vi "Master Target.vi"() -> ()   [LabVIEW 2011]
uses:
  Common/controls/Grips Buttons.ctl
  Common/classes/PXI/PXI.lvclass
  Common/classes/GripsMaster/GripsMaster.lvclass
  Common/controls/Task Definition.ctl
  Common/controls/Task Types.ctl
  Common/labview_msgs/sensor_msgs/JointState.ctl
panel:
  in  "Slave IP":string="138.100.76.41"
  out "UDP Status":errorcluster
  in  "Write Port":u16=5555
  out "Grips Buttons":T1
  in  "Stop":bool
  out "Controller Status":errorcluster
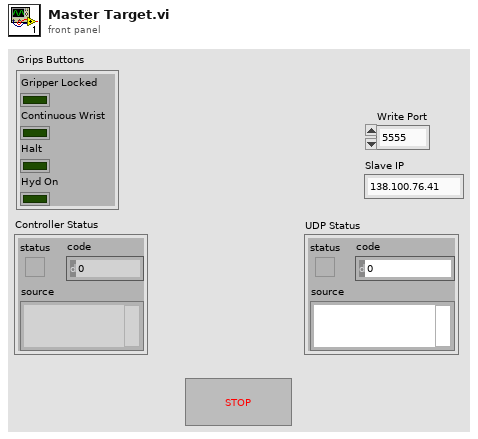
[diagram p1: front panel]
types:
  T1 = typedef "Grips Buttons.ctl" = cluster{"Gripper Locked":bool, "Continuous Wrist":bool, "Halt":bool, "Hyd On":bool}
  T2 = typedef "Task Definition.ctl" = cluster{"task_type":T3, "names":string[], "physical channels":tag, "min_value":dbl, "max_value":dbl, "task_number":i32}
  T3 = typedef "Task Types.ctl" = enum16{"Analog Input", "Analog Output", "Digital Input", "Digital Output"}
  T4 = typedef "Digital Values.ctl" = cluster{"names":string[], "values":bool[]}
  T5 = typedef "Analog Values.ctl" = cluster{"names":string[], "values":dbl[]}
  T6 = enum16{"big-endian, network order", "native, host order", "little-endian"}
  T7 = typedef "JointState.ctl" = cluster{"header":cluster{"seq":u32, "stamp":cluster{"sec":i32, "nsec":i32}, "frame_id":string}, "name":string[], "position":dbl[], "velocity":dbl[], "effort":dbl[]}
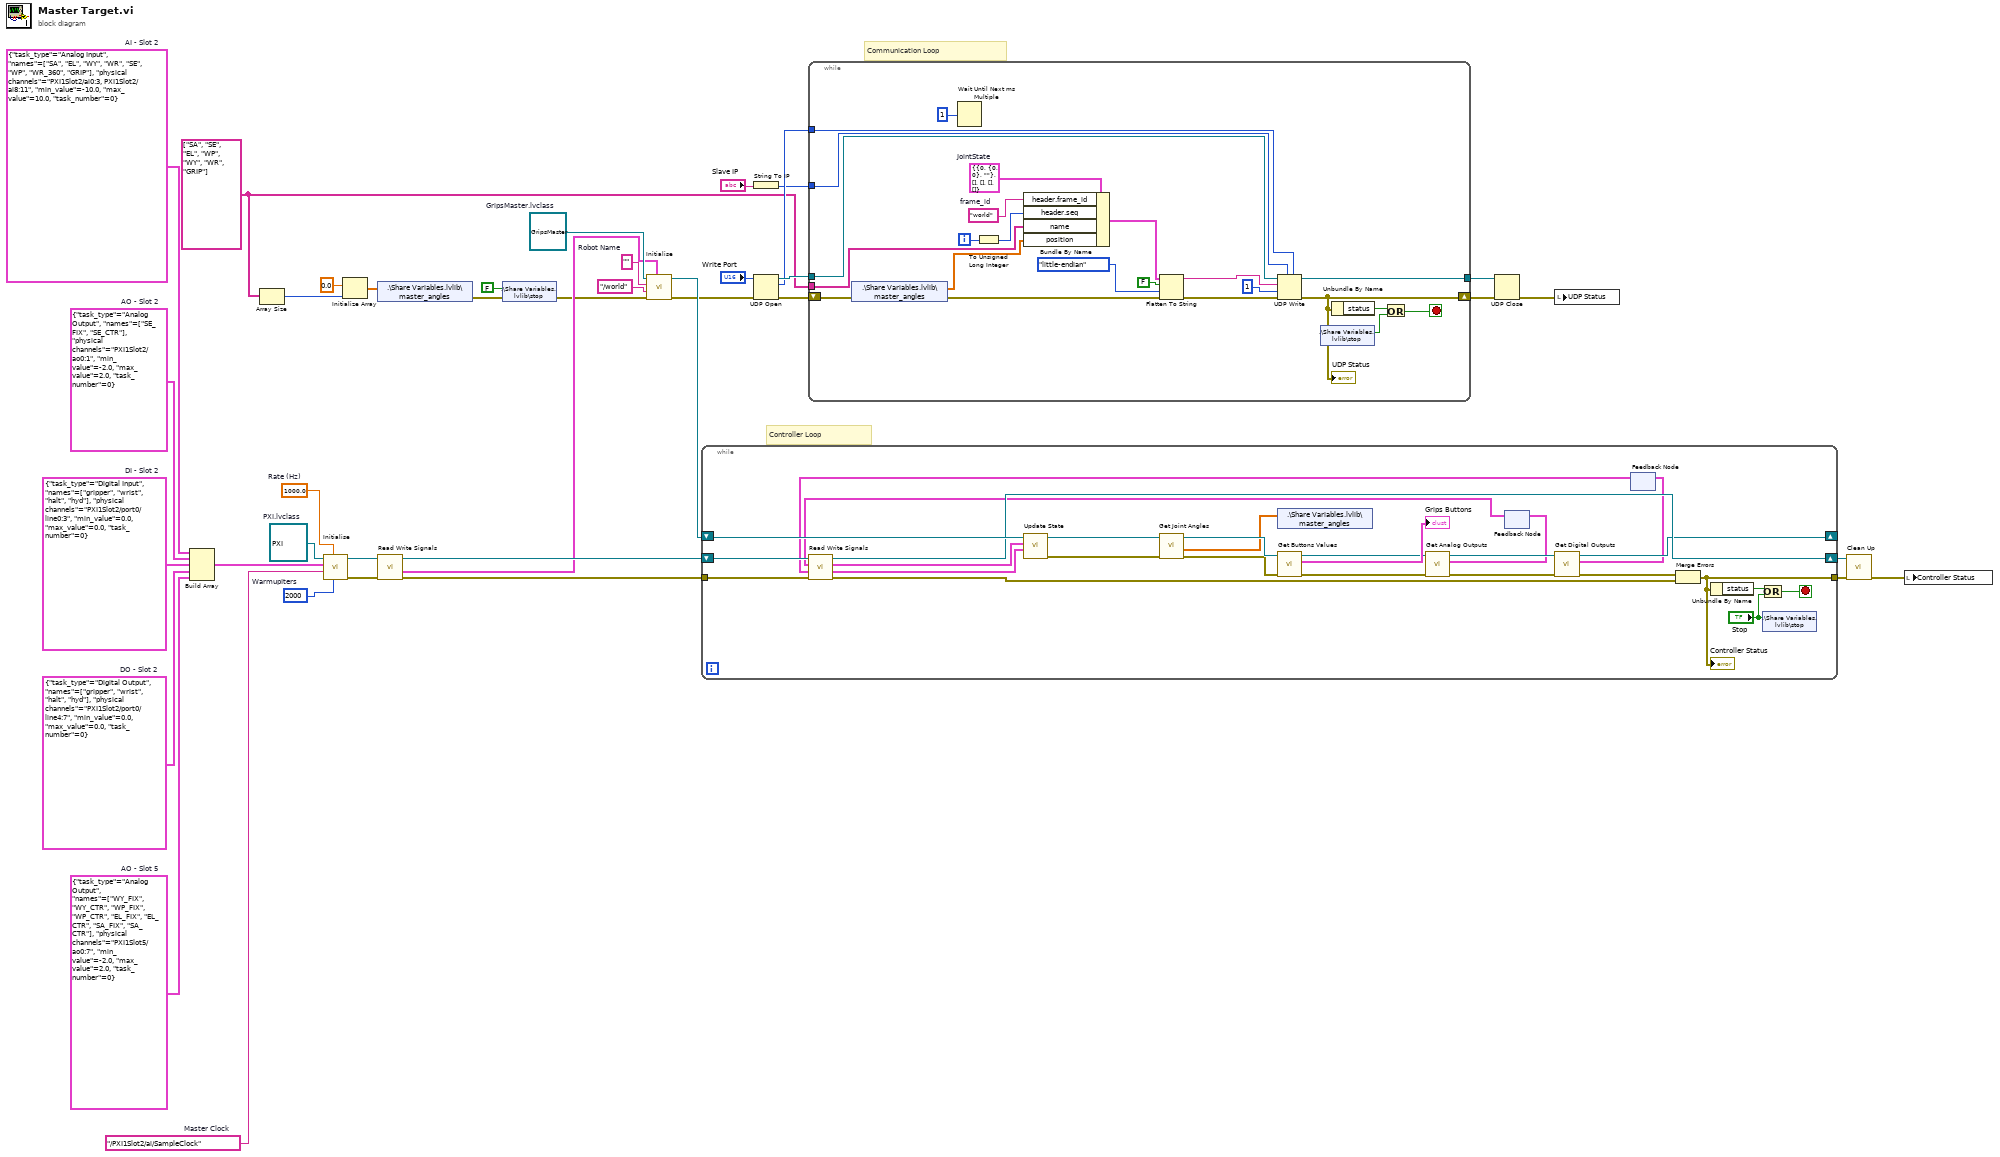
[diagram p0: block diagram]
diagram:
  w4 = string[] ["SA", "SE", "EL", "WP", "WY", "WR", "GRIP"] ("names")
  w5 = T2 {"task_type"=enum."Analog Output", "names"=["WY_FIX", "WY_CTR", "WP_FIX", "WP_CTR", "EL_FIX", "EL_CTR", "SA_FIX", "SA_CTR"], "physical channels"="PXI1Slot5/ao0:7", "min_value"=-2.0, "max_value"=2.0, "task_number"=0}  # AO - Slot 5
  w7 = T2 {"task_type"=enum."Digital Input", "names"=["gripper", "wrist", "halt", "hyd"], "physical channels"="PXI1Slot2/port0/line0:3", "min_value"=0.0, "max_value"=0.0, "task_number"=0}  # DI - Slot 2
  w6 = T2 {"task_type"=enum."Digital Output", "names"=["gripper", "wrist", "halt", "hyd"], "physical channels"="PXI1Slot2/port0/line4:7", "min_value"=0.0, "max_value"=0.0, "task_number"=0}  # DO - Slot 2
  w8 = T2 {"task_type"=enum."Analog Output", "names"=["SE_FIX", "SE_CTR"], "physical channels"="PXI1Slot2/ao0:1", "min_value"=-2.0, "max_value"=2.0, "task_number"=0}  # AO - Slot 2
  w9 = T2 {"task_type"=enum."Analog Input", "names"=["SA", "EL", "WY", "WR", "SE", "WP", "WR_360", "GRIP"], "physical channels"="PXI1Slot2/ai0:3, PXI1Slot2/ai8:11", "min_value"=-10.0, "max_value"=10.0, "task_number"=0}  # AI - Slot 2
  w31 = ""  # Robot Name
  w32 = refnum<class "GripsMaster.lvclass"> refnum  # GripsMaster.lvclass
  w38 = 1000.0  # Rate (Hz)
  w35 = u32 2000  # WarmupIters
  w37 = tag "/PXI1Slot2/ai/SampleClock"  # Master Clock
  w39 = refnum<class "PXI.lvclass"> refnum  # PXI.lvclass
  # "Communication Loop"
  # "Controller Loop"
  n1 = Build Array(w9, w8, w7, w6, w5) -> (w36:T2[])
  n2 = Array Size(array=w4) -> (size(s)=w3:i32)
  n3 = call "Initialise.vi"("WarmupIters"=w35, "Rate (Hz)"=w38, "Master Clock"=w37, "Tasks Info"=w36, "PXI in"=w39) -> ("error out"=w33:errorcluster, "PXI out"=w34:refnum<class "PXI.lvclass">)  [unwired: 5 in]
  n4 = Initialize Array(0.0 ("element"), w3) -> (w11:dbl[])
  n5 = shared-variable ".\\Share Variables.lvlib\\master_angles"(w11) -> (error out=w15:errorcluster)  [unwired: 1 in]
  n6 = call "Read Write Signals.vi"("error in (no error)"=w33, "PXI in"=w34) -> ("error out"=w28:errorcluster, "Digital Inputs"=w24:T4, "PXI out"=w29:refnum<class "PXI.lvclass">)  [unwired: 6 in, 1 out]
  n7 = shared-variable ".\\Share Variables.lvlib\\stop"(FALSE ("stop"), error in=w15) -> (error out=w13:errorcluster)
  n8 = call "Initialise.vi"("Initial DI"=w24, "error in (no error)"=w13, "Robot Frame"="/world", "Robot Name"=w31, "Master in"=w32) -> ("error out"=w10:errorcluster, "Master out"=w25:refnum<class "GripsMaster.lvclass">)  [unwired: 5 in]
  n9 = while {
    tunnel: w28 -> [w62]
    tunnel: [w55] -> w26
    shift-right: [w61] -> w27
    shift-left: w29 -> [w63]
    shift-right: [w46] -> _
    shift-left: w25 -> [w66]
    stop <- w57 stop-if-true
    n10 = feedback #1() -> (w42:T5)  [unwired: 1 in]
    n11 = feedback #2() -> (w40:T4)  [unwired: 1 in]
    n12 = call "Read Write Signals.vi"("error in (no error)"=w62, "Digital Outputs"=w40, "Analog Outputs"=w42, "PXI in"=w63) -> ("error out"=w60:errorcluster, "Digital Inputs"=w58:T4, "Analog Inputs"=w59:T5, "PXI out"=w61:refnum<class "PXI.lvclass">)  [unwired: 4 in]
    n13 = call "Update State.vi"("Digital Inputs"=w58, "Analog Inputs"=w59, "GripsMaster in"=w66) -> ("error out"=w64:errorcluster, "GripsMaster out"=w65:refnum<class "GripsMaster.lvclass">)  [unwired: 7 in]
    n14 = call "Get Joint Angles.vi"("error in (no error)"=w64, "GripsMaster in"=w65) -> ("error out"=w53:errorcluster, "simulator_angles"=w50:dbl[], "GripsMaster out"=w54:refnum<class "GripsMaster.lvclass">)  [unwired: 6 in, 1 out]
    n15 = shared-variable ".\\Share Variables.lvlib\\master_angles"(w50) -> ()  [unwired: 1 in, 1 out]
    n16 = call "Get Buttons Values.vi"("error in (no error)"=w53, "GripsMaster in"=w54) -> ("error out"=w44:errorcluster, "Grips Buttons"=→"Grips Buttons":T1, "GripsMaster out"=w45:refnum<class "GripsMaster.lvclass">)  [unwired: 7 in]
    n17 = call "Get Analog Outputs.vi"("error in (no error)"=w44, "GripsMaster in"=w45) -> ("error out"=w48:errorcluster, "Analog Values"=w43:T5, "GripsMaster out"=w49:refnum<class "GripsMaster.lvclass">)  [unwired: 7 in]
    n18 = feedback-in #1(w43) -> ()
    n19 = call "Get Digital Outputs.vi"("error in (no error)"=w48, "GripsMaster in"=w49) -> ("error out"=w47:errorcluster, "Digital Values"=w41:T4, "GripsMaster out"=w46:refnum<class "GripsMaster.lvclass">)  [unwired: 7 in]
    n20 = feedback-in #2(w41) -> ()
    n21 = Merge Errors(w47, w60) -> (w55:errorcluster)
    "Controller Status" <- w55
    n22 = Unbundle By Name(w55) -> ("status"=w56:bool)
    n23 = Or(x=w56, y="Stop") -> (x .or. y?=w57:bool)
    n24 = shared-variable ".\\Share Variables.lvlib\\stop"("Stop") -> ()  [unwired: 1 in, 1 out]
  }
  n25 = String To IP(1:"Slave IP") -> (0:w16:u32)
  n26 = UDP Open(8:w10, 11:"Write Port") -> (port=w21:refnum<k16>, 0:w20:errorcluster, 2:w18:u16)  [unwired: 3 out]
  n27 = while {
    tunnel: [w83] -> w22
    tunnel: w21 -> [w82]
    tunnel: w18 -> [w81]
    shift-right: [w80] -> w19
    shift-left: w20 -> [w68]
    tunnel: w4 -> [w73]
    tunnel: w16 -> [w72]
    i -> [w84]
    stop <- w78 stop-if-true
    w71 = T7 {"header"={"seq"=0, "stamp"={"sec"=0, "nsec"=0}, "frame_id"=""}, "name"=[], "position"=[], "velocity"=[], "effort"=[]}  # JointState
    w75 = "world"  # frame_id
    n28 = shared-variable ".\\Share Variables.lvlib\\master_angles"(error in=w68) -> (w69:dbl[], error out=w67:errorcluster)
    n29 = Wait Until Next ms Multiple(millisecond multiple=u32 1 ("milliseconds to wait")) -> ()  [unwired: 1 out]
    n30 = To Unsigned Long Integer(number=w84) -> (unsigned 32bit integer=w76:u32)
    n31 = Bundle By Name(cluster=w71, "header.frame_id"=w75, "header.seq"=w76, "name"=w73, "position"=w69) -> (w85:T7)
    n32 = Flatten To String(anything=w85, prepend array or string size? (T)=FALSE, byte order (0:big-endian, network order)=T6."little-endian" ("Byte order"), error in (no error)=w67) -> (data string=w88:string, error out=w86:errorcluster)  [unwired: 1 out]
    n33 = UDP Write(address=w72, port or service name=w81, connection ID=w82, data in=w88, 8:w86, 9:1 ("timeout ms (25000)")) -> (error out=w80:errorcluster, 3:w83:refnum<k16>)
    "UDP Status" <- w80
    n34 = shared-variable ".\\Share Variables.lvlib\\stop"() -> (w70:bool)  [unwired: 1 in, 1 out]
    n35 = Unbundle By Name(w80) -> ("status"=w79:bool)
    n36 = Or(x=w79, y=w70) -> (x .or. y?=w78:bool)
  }
  n37 = UDP Close(connection ID=w22, 8:w19) -> (error out=w2:errorcluster)  [unwired: 1 out]
  n38 = local write "UDP Status"(w2) -> ()
  n39 = call "Clean Up.vi"("error in (no error)"=w26, "PXI in"=w27) -> ("error out"=w1:errorcluster)  [unwired: 8 in, 1 out]
  n40 = local write "Controller Status"(w1) -> ()
